vi "duration in sec.vi"(11 "input time mm:ss":string[](array[string])) -> (3 "total in sec":i32[](array[numeric]))   [LabVIEW 2017]
panel:
  out "sec":i32[](array[numeric])
  out "min":i32[](array[numeric])
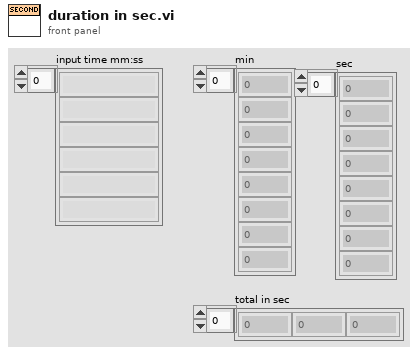
[diagram p1: front panel]
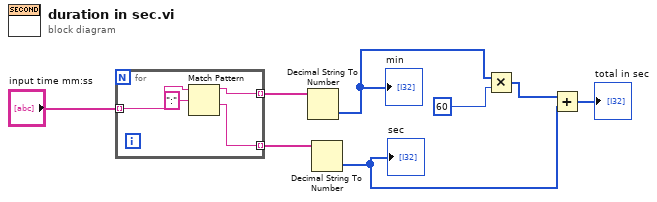
[diagram p0: block diagram]
diagram:
  n1 = for {
    tunnel: "input time mm:ss" -> [w11] mode=indexing
    tunnel: [w10] -> w2 mode=indexing
    tunnel: [w9] -> w3 mode=indexing
    n2 = Match Pattern(string=w11, regular expression=":") -> (before substring=w10:string, after substring=w9:string)  [unwired: 1 in, 2 out]
  }
  n3 = Decimal String To Number(string=w2) -> (number=w4:i32[])  [unwired: 2 in, 1 out]
  "min" <- w4
  n4 = Decimal String To Number(string=w3) -> (number=w7:i32[])  [unwired: 2 in, 1 out]
  "sec" <- w7
  n5 = Multiply(x=w4, y=60 ("result string")) -> (x*y=w5:i32[])
  n6 = Add(x=w5, y=w7) -> (x+y=→"total in sec":i32[])
